vi "cambioZ.vi"(9 "DISTANCIA":dbl, 11 "TARGET":dbl) -> (2 "CAMBIO Z":dbl)   [LabVIEW 2018]
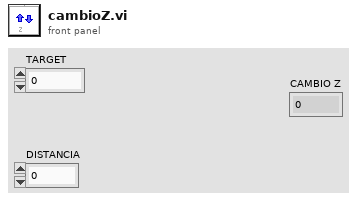
[diagram p1: front panel]
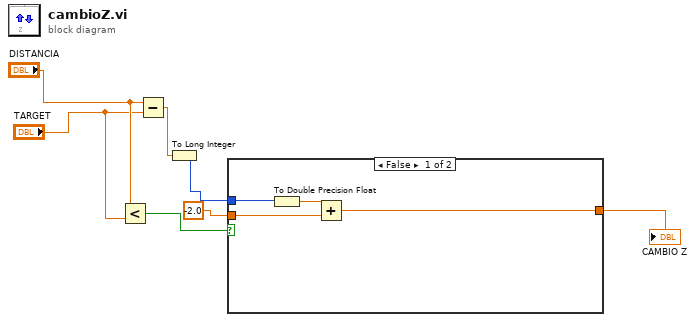
[diagram p0: block diagram]
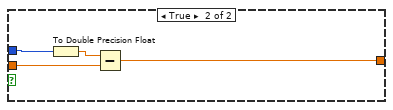
[diagram p2: hidden frame]
diagram:
  n1 = Less?(x="DISTANCIA", y="TARGET") -> (x < y?=w4:bool)
  n2 = Subtract(x="DISTANCIA", y="TARGET") -> (x-y=w7:dbl)
  n3 = To Long Integer(number=w7) -> (32bit integer=w3:i32)
  n4 = case shown="False" w4 {
    tunnel: w3 -> [w11 w15]
    tunnel: [w8 w13] -> w2
    tunnel: -2.0 ("y") -> [w9 w12]
    frame False {
      n5 = To Double Precision Float(number=w11) -> (double precision float=w10:dbl)
      n6 = Add(x=w10, y=w9) -> (x+y=w8:dbl)
    }
    frame True {
      n7 = To Double Precision Float(number=w15) -> (double precision float=w14:dbl)
      n8 = Subtract(x=w14, y=w12) -> (x-y=w13:dbl)
    }
  }
  "CAMBIO Z" <- w2
